vi "Lambda Genesys Engine.vi"() -> ()   [LabVIEW 2011, in "Lambda Genesys2 Custom Device.lvlib"]
uses:
  Lambda Genesys2 Custom Device.lvlib
  <vilib>/NI Veristand/Custom Device API/Custom Device Item Ref.ctl
  <vilib>/NI Veristand/Custom Device API/Custom Device Channel Type.ctl
  Lambda Genesys Device Properties.vi
  <vilib>/NI Veristand/Custom Device API/Get Item Property (I32).vi
  <vilib>/NI Veristand/Custom Device API/Get Item Property (String).vi
  <vilib>/NI Veristand/Custom Device API/Custom Device API.lvlib
panel:
  in  "Status Notifier":refnum<notifier>
  in  "Device Reference":T1=18446744073709551615 format="%.0x"
  in  "Device Inputs FIFO":refnum<k33>
  in  "Device Outputs FIFO":refnum<k33>
  # "Lambda Genesys Custom Device Engine"
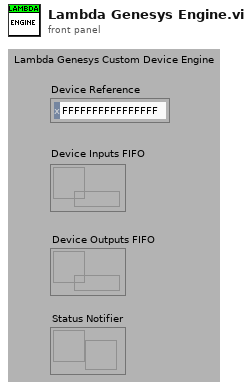
[diagram p1: front panel]
types:
  T1 = typedef "Custom Device API.lvlib/Custom Device Item Ref.ctl" = u64
  T2 = cluster{"Output Indices":i32[], "Input Indices":i32[], "Device Reference":T1, "Output Data":dbl[], "Input Data":dbl[], "Instr.Handle":refnum<visa-resource-name>, "GEN Addr":i16, "Device Outputs FIFO":refnum<k33>, "Device Inputs FIFO":refnum<k33>, "Previous Inputs":dbl[], "Device Error":errorcluster, "Status Notifier":refnum<notifier>}
  T3 = typedef "Custom Device API.lvlib/Custom Device Channel Type.ctl" = enum16{"Input", "Output"}
  T4 = typedef "Custom Device API.lvlib/Custom Device Item Info.ctl" = cluster{"Name":string, "Is Channel":bool, "GUID":string}
  T5 = typedef "Custom Device API.lvlib/Custom Device Channel.ctl" = cluster{"Type":T3, "Units":string, "Default Value":dbl, "Faultable":bool, "Scalable":bool}
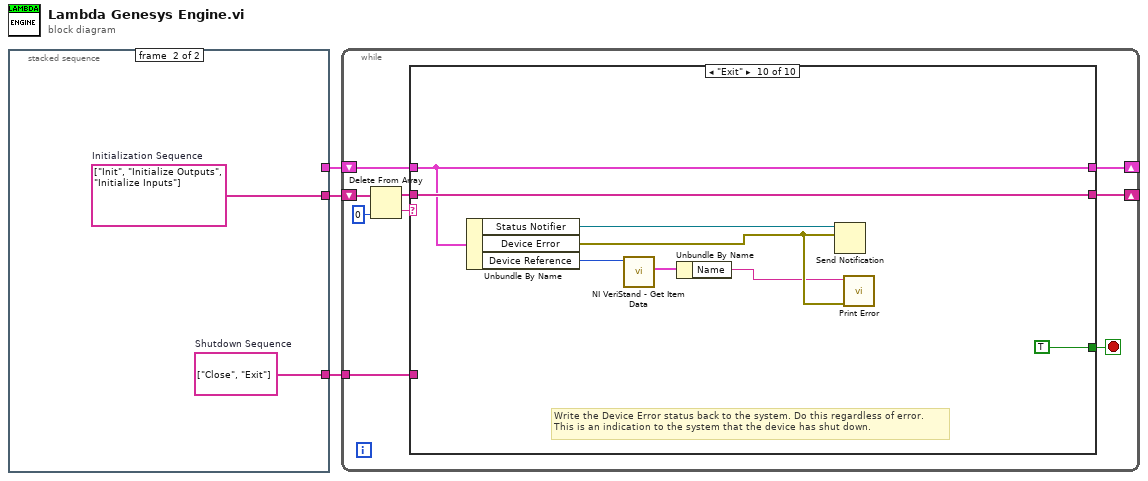
[diagram p0: block diagram]
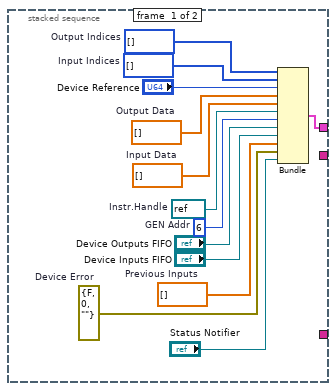
[diagram p2: hidden frame]
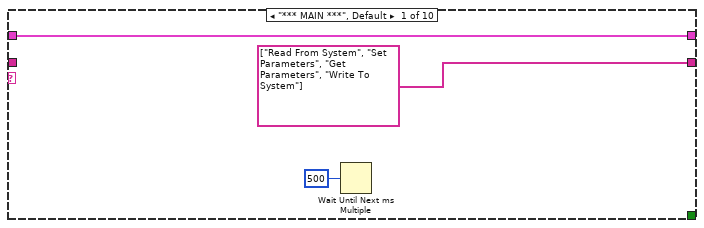
[diagram p3: hidden frame]
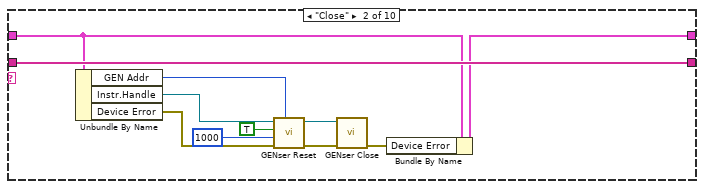
[diagram p4: hidden frame]
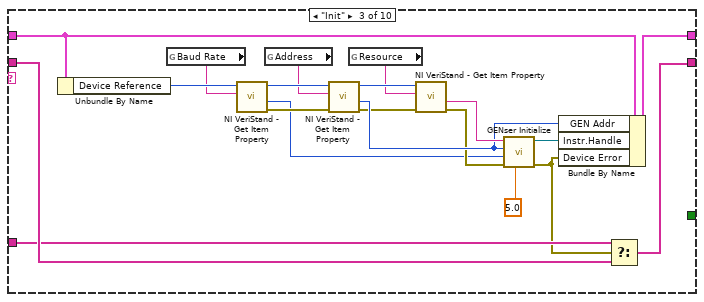
[diagram p5: hidden frame]
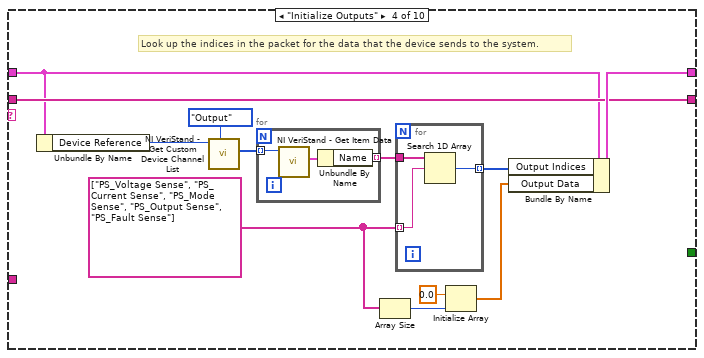
[diagram p6: hidden frame]
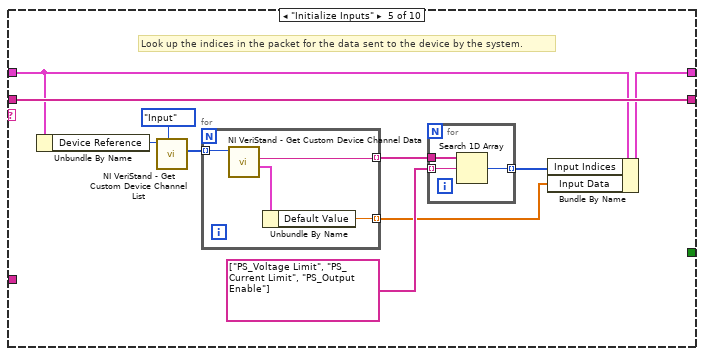
[diagram p7: hidden frame]
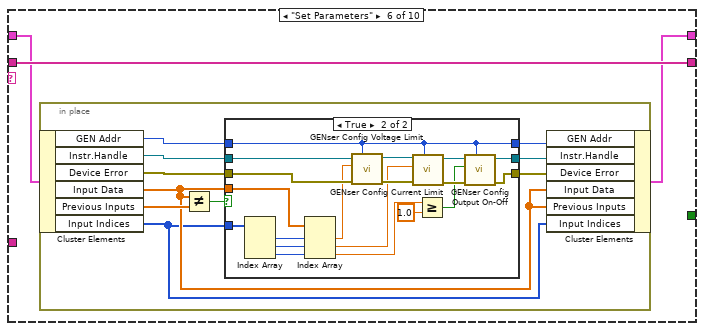
[diagram p8: hidden frame]
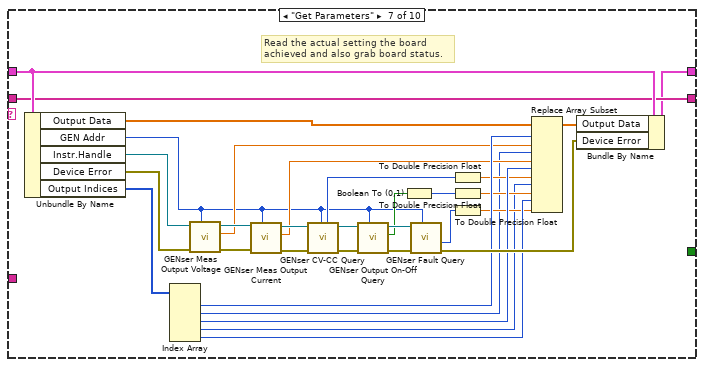
[diagram p10: hidden frame]
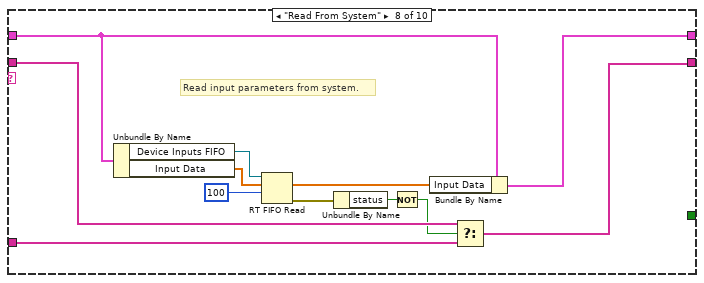
[diagram p11: hidden frame]
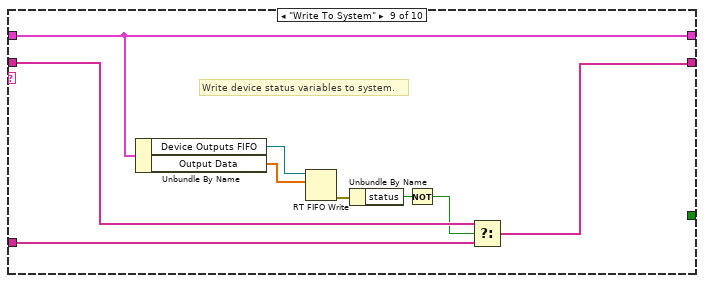
[diagram p12: hidden frame]
diagram:
  n1 = stacked-sequence {
    tunnel: [_ w18] -> w3
    tunnel: [w14 _] -> w2
    tunnel: [_ w17] -> w1
    frame #0 {
      w5 = i32[] []  # Output Indices
      w6 = i32[] []  # Input Indices
      w9 = dbl[] []  # Previous Inputs
      w7 = errorcluster {"status"=FALSE, "code"=0, "source"=""}  # Device Error
      w10 = dbl[] []  # Input Data
      w11 = dbl[] []  # Output Data
      w15 = i16 6  # GEN Addr
      w16 = refnum<visa-resource-name> refnum  # Instr.Handle
      n2 = Bundle("Output Indices"=w5, "Input Indices"=w6, "Device Reference"="Device Reference", "Output Data"=w11, "Input Data"=w10, "Instr.Handle"=w16, "GEN Addr"=w15, "Device Outputs FIFO"="Device Outputs FIFO", "Device Inputs FIFO"="Device Inputs FIFO", "Previous Inputs"=w9, "Device Error"=w7, "Status Notifier"="Status Notifier") -> (w14:T2)  [unwired: 1 out]
    }
    frame #1 {
      w17 = string[] ["Close", "Exit"]  # Shutdown Sequence
      w18 = string[] ["Init", "Initialize Outputs", "Initialize Inputs"]  # Initialization Sequence
    }
  }
  n3 = while {
    shift-right: [w23] -> _
    shift-left: w3 -> [w27]
    shift-right: [w21] -> _
    shift-left: w2 -> [w22]
    tunnel: w1 -> [w19]
    stop <- w20 stop-if-true
    n4 = Delete From Array(array=w27, index=0) -> (deleted portion=w26:string, array with subset deleted=w24:string[])  [unwired: 1 in]
    n5 = case shown="\"Exit\"" w26 {
      tunnel: w24 -> [_ w41 w50 w72 w89 w99 w138 w175 w179 w192]
      tunnel: [string[] ["Read From System", "Set Parameters", "Get Parameters", "Write To System"] w41 w53 w72 w89 w99 w138 w170 w181 w192] -> w23
      tunnel: w22 -> [w28 w32 w54 w66 w84 w98 w158 w174 w184 w190]
      tunnel: [w28 w31 w51 w73 w83 w97 w137 w172 w184 w190] -> w21
      tunnel: [_ _ _ _ _ _ _ _ _ TRUE] -> w20
      tunnel: w19 -> [_ _ w47 _ _ _ _ w166 w177 _]
      frame "*** MAIN ***", Default {
        n6 = Wait Until Next ms Multiple(millisecond multiple=u32 500 ("Timeout (0)")) -> ()  [unwired: 1 out]
      }
      frame "Close" {
        n7 = Unbundle By Name(w32) -> ("GEN Addr"=w37:i16, "Instr.Handle"=w38:refnum<visa-resource-name>, "Device Error"=w34:errorcluster)
        n8 = call <instrlib>:"GENser Reset.vi"("GEN Addr"=w37, "error"=w34, "Settle (0 mS)"=u32 1000, "Reset (T)"=TRUE, "VISA"=w38) -> ("error out"=w39:errorcluster, "VISA out"=w40:refnum<visa-resource-name>)  [unwired: 5 out]
        n9 = call <instrlib>:"GENser Close.vi"("error"=w39, "VISA name"=w40) -> ("error out"=w33:errorcluster)  [unwired: 9 out]
        n10 = Bundle By Name(cluster=w32, "Device Error"=w33) -> (w31:T2)
      }
      frame "Init" {
        n11 = Unbundle By Name(w54) -> ("Device Reference"=w59:T1)
        n12 = global read "Lambda Genesys Device Properties.vi" "Baud Rate"() -> (w43:string)
        n13 = call-poly <vilib>:"NI VeriStand - Get Item Property.vi"("Property Name"=w43, "Item Ref in"=w59) -> ("error out"=w56:errorcluster, "Value"=w42:i32, "Item Ref out"=w57:T1)  [unwired: 2 in, 5 out]
        n14 = global read "Lambda Genesys Device Properties.vi" "Address"() -> (w45:string)
        n15 = call-poly <vilib>:"NI VeriStand - Get Item Property.vi"("error in (no error)"=w56, "Property Name"=w45, "Item Ref in"=w57) -> ("error out"=w44:errorcluster, "Value"=w60:i32, "Item Ref out"=w55:T1)  [unwired: 1 in, 5 out]
        n16 = global read "Lambda Genesys Device Properties.vi" "Resource"() -> (w48:string)
        n17 = call-poly <vilib>:"NI VeriStand - Get Item Property.vi"("error in (no error)"=w44, "Property Name"=w48, "Item Ref in"=w55) -> ("error out"=w58:errorcluster, "Value"=w61:string)  [unwired: 1 in, 6 out]
        n18 = call <instrlib>:"GENser Initialize.vi"("Timeout (3 sec)"=5.0, "error in (no error)"=w58, "BAUD"=w42, "GEN Addr"=w60, "VISA name"=w61) -> ("error out"=w46:errorcluster, "VISA out"=w49:refnum<visa-resource-name>)  [unwired: 2 in, 3 out]
        n19 = Bundle By Name(cluster=w54, "GEN Addr"=w60, "Instr.Handle"=w49, "Device Error"=w46) -> (w51:T2)
        n20 = Select(t=w47, s=w46, f=w50) -> (s? t:f=w53:string[])
      }
      frame "Initialize Outputs" {
        w65 = string[] ["PS_Voltage Sense", "PS_Current Sense", "PS_Mode Sense", "PS_Output Sense", "PS_Fault Sense"]
        # "Look up the indices in the packet for the data that the device sends to the system."
        n21 = Unbundle By Name(w66) -> ("Device Reference"=w70:T1)
        n22 = call <vilib>:"NI VeriStand - Get Custom Device Channel List.vi"("Channel Type"=Custom_Device_Channel_Type."Output", "Device Ref in"=w70) -> ("Specified Channel Ref List"=w69:T1[])  [unwired: 1 in, 8 out]
        n23 = for {
          tunnel: w69 -> [w79] mode=indexing
          tunnel: [w77] -> w68 mode=indexing
          n24 = call <vilib>:"NI VeriStand - Get Item Data.vi"("Item Ref in"=w79) -> ("Item Info"=w78:T4)  [unwired: 1 in, 9 out]
          n25 = Unbundle By Name(w78) -> ("Name"=w77:string)
        }
        n26 = Array Size(array=w65) -> (size(s)=w64:i32)
        n27 = for {
          tunnel: w68 -> [w76]
          tunnel: w65 -> [w75] mode=indexing
          tunnel: [w74] -> w67 mode=indexing
          n28 = Search 1D Array(1D array=w76, element=w75) -> (index of element=w74:i32)  [unwired: 1 out]
        }
        n29 = Initialize Array(0.0 ("element"), w64) -> (w62:dbl[])
        n30 = Bundle By Name(cluster=w66, "Output Indices"=w67, "Output Data"=w62) -> (w73:T2)
      }
      frame "Initialize Inputs" {
        # "Look up the indices in the packet for the data sent to the device by the system."
        n31 = Unbundle By Name(w84) -> ("Device Reference"=w87:T1)
        n32 = call <vilib>:"NI VeriStand - Get Custom Device Channel List.vi"("Channel Type"=Custom_Device_Channel_Type."Input", "Device Ref in"=w87) -> ("Specified Channel Ref List"=w86:T1[])  [unwired: 1 in, 8 out]
        n33 = for {
          tunnel: w86 -> [w96] mode=indexing
          tunnel: [w95] -> w85 mode=indexing
          tunnel: [w93] -> w80 mode=indexing
          n34 = call <vilib>:"NI VeriStand - Get Custom Device Channel Data.vi"("Channel Ref in"=w96) -> ("Channel"=w94:T5, "Channel Name"=w95:string)  [unwired: 5 in, 4 out]
          n35 = Unbundle By Name(w94) -> ("Default Value"=w93:dbl)
        }
        n36 = for {
          tunnel: w85 -> [w92]
          tunnel: string[] ["PS_Voltage Limit", "PS_Current Limit", "PS_Output Enable"] -> [w91] mode=indexing
          tunnel: [w90] -> w81 mode=indexing
          n37 = Search 1D Array(1D array=w92, element=w91) -> (index of element=w90:i32)  [unwired: 1 out]
        }
        n38 = Bundle By Name(cluster=w84, "Input Indices"=w81, "Input Data"=w80) -> (w83:T2)
      }
      frame "Set Parameters" {
        n39 = in-place {
          n40 = in-place-cluster #1(w98) -> ("GEN Addr"=w108:i16, "Instr.Handle"=w106:refnum<visa-resource-name>, "Device Error"=w101:errorcluster, "Input Data"=w103:dbl[], "Previous Inputs"=w104:dbl[], "Input Indices"=w102:i32[])
          n41 = Not Equal?(x=w103, y=w104) -> (x != y?=w109:bool)
          n42 = case shown="True" w109 {
            tunnel: w106 -> [w111 w122]
            tunnel: [w111 w127] -> w105
            tunnel: w108 -> [w112 w123]
            tunnel: [w112 w123] -> w107
            tunnel: w103 -> [_ w121]
            tunnel: w102 -> [_ w117]
            tunnel: w101 -> [w110 w131]
            tunnel: [w110 w113] -> w100
            frame False {
              # "Update settings only if setpoint has changed."
            }
            frame True {
              n43 = Index Array(array=w117) -> (element #1=w116:i32, element #2=w115:i32, element #3=w114:i32)  [unwired: 3 in]
              n44 = Index Array(array=w121, index #1=w116, index #2=w115, index #3=w114) -> (element #1=w120:dbl, element #2=w119:dbl, element #3=w118:dbl)
              n45 = call <instrlib>:"GENser Config Voltage Limit.vi"("GEN Addr"=w123, "error"=w131, "Volt Limit"=w120, "VISA"=w122) -> ("error out"=w130:errorcluster, "VISA out"=w129:refnum<visa-resource-name>)  [unwired: 1 in, 5 out]
              n46 = call <instrlib>:"GENser Config Current Limit.vi"("GEN Addr"=w123, "error"=w130, "Current Limit"=w119, "VISA"=w129) -> ("error out"=w126:errorcluster, "VISA out"=w128:refnum<visa-resource-name>)  [unwired: 1 in, 5 out]
              n47 = Greater Or Equal?(x=w118, y=1.0) -> (x >= y?=w124:bool)
              n48 = call <instrlib>:"GENser Config Output On-Off.vi"("GEN Addr"=w123, "error"=w126, "Output ON"=w124, "VISA"=w128) -> ("error out"=w113:errorcluster, "VISA out"=w127:refnum<visa-resource-name>)  [unwired: 1 in, 5 out]
            }
          }
          n49 = in-place-cluster #1("GEN Addr"=w107, "Instr.Handle"=w105, "Device Error"=w100, "Input Data"=w103, "Previous Inputs"=w103, "Input Indices"=w102) -> (w97:T2)
        }
      }
      frame "Get Parameters" {
        # "Read the actual setting the board achieved and also grab board status."
        n50 = Unbundle By Name(w158) -> ("Output Data"=w152:dbl[], "GEN Addr"=w136:i16, "Instr.Handle"=w157:refnum<visa-resource-name>, "Device Error"=w133:errorcluster, "Output Indices"=w132:i32[])
        n51 = Index Array(array=w132) -> (element #1=w162:i32, element #2=w135:i32, element #3=w161:i32, element #4=w134:i32, element #5=w160:i32)  [unwired: 5 in]
        n52 = call <instrlib>:"GENser Meas Output Voltage.vi"("GEN Addr"=w136, "error"=w133, "VISA"=w157) -> ("error out"=w155:errorcluster, "Output Voltage"=w151:dbl, "VISA out"=w156:refnum<visa-resource-name>)  [unwired: 6 out]
        n53 = call <instrlib>:"GENser Meas Output Current.vi"("GEN Addr"=w136, "error"=w155, "VISA"=w156) -> ("error out"=w153:errorcluster, "Output Current"=w143:dbl, "VISA out"=w154:refnum<visa-resource-name>)  [unwired: 6 out]
        n54 = call <instrlib>:"GENser CV-CC Query.vi"("GEN Addr"=w136, "error"=w153, "VISA"=w154) -> ("error out"=w149:errorcluster, "VISA out"=w148:refnum<visa-resource-name>, "Mode"=w150:enum16{"OFF", "CV", "CC"})  [unwired: 6 out]
        n55 = call <instrlib>:"GENser Output On-Off Query.vi"("GEN Addr"=w136, "error"=w149, "VISA"=w148) -> ("error out"=w145:errorcluster, "Output ON"=w146:bool, "VISA out"=w159:refnum<visa-resource-name>)  [unwired: 6 out]
        n56 = Boolean To (0,1)(Boolean=w146) -> (0, 1=w147:i16)
        n57 = call <instrlib>:"GENser Fault Query.vi"("GEN Addr"=w136, "error"=w145, "VISA"=w159) -> ("error out"=w163:errorcluster, "Fault Register"=w144:u8)  [unwired: 7 out]
        n58 = To Double Precision Float(number=w150) -> (double precision float=w140:dbl)
        n59 = To Double Precision Float(number=w147) -> (double precision float=w141:dbl)
        n60 = To Double Precision Float(number=w144) -> (double precision float=w142:dbl)
        n61 = Replace Array Subset(array=w152, new element #1=w151, index #1=w162, new element #2=w143, index #2=w135, new element #3=w140, index #3=w161, new element #4=w141, index #4=w134, new element #5=w142, index #5=w160) -> (w139:dbl[])
        n62 = Bundle By Name(cluster=w158, "Output Data"=w139, "Device Error"=w163) -> (w137:T2)
      }
      frame "Read From System" {
        # "Read input parameters from system."
        n63 = Unbundle By Name(w174) -> ("Device Inputs FIFO"=w164:refnum<k33>, "Input Data"=w173:dbl[])
        n64 = RT FIFO Read(0:w164, 1:w173, 2:100 ("timeout in ms (0)")) -> (9:w171:dbl[], 11:w169:errorcluster)  [unwired: 1 in, 3 out]
        n65 = Unbundle By Name(w169) -> ("status"=w168:bool)
        n66 = Not(x=w168) -> (.not. x?=w167:bool)
        n67 = Bundle By Name(cluster=w174, "Input Data"=w171) -> (w172:T2)
        n68 = Select(t=w175, s=w167, f=w166) -> (s? t:f=w170:string[])
      }
      frame "Write To System" {
        # "Write device status variables to system."
        n69 = Unbundle By Name(w184) -> ("Device Outputs FIFO"=w176:refnum<k33>, "Output Data"=w183:dbl[])
        n70 = RT FIFO Write(0:w176, 1:w183) -> (11:w182:errorcluster)  [unwired: 2 in, 4 out]
        n71 = Unbundle By Name(w182) -> ("status"=w180:bool)
        n72 = Not(x=w180) -> (.not. x?=w178:bool)
        n73 = Select(t=w179, s=w178, f=w177) -> (s? t:f=w181:string[])
      }
      frame "Exit" {
        # "Write the Device Error status back to the system. Do this regardless of error.\nThis is an indication to the system that the device has shut down."
        n74 = Unbundle By Name(w190) -> ("Status Notifier"=w189:refnum<notifier>, "Device Error"=w188:errorcluster, "Device Reference"=w187:T1)
        n75 = call <vilib>:"NI VeriStand - Get Item Data.vi"("Item Ref in"=w187) -> ("Item Info"=w186:T4)  [unwired: 7 in, 3 out]
        n76 = Unbundle By Name(w186) -> ("Name"=w185:string)
        n77 = Send Notification(notification=w188, notifier=w189) -> ()  [unwired: 1 in, 2 out]
        n78 = call "Print Error.vi"("error out"=w188, "Your code's public name"=w185) -> ()  [unwired: 9 in]
      }
    }
  }
